vi "P4CMDSub Verify File Status for CheckIn.vi"(6 "operation message":string, 8 "error in (no error)":errorcluster, 10 "files":path[](array[path]), 11 "source control reference in":T1) -> (0 "error out":errorcluster, 2 "files (depot format)":string[](array[string]), 3 "source control reference out":T1, 5 "active changelist":string)   [LabVIEW 2017, in "NI_SCC_P4CMD.lvlib"]
uses:
  <vilib>/SourceControl/Providers/P4CMD/NI_SCC_P4CMD.lvlib
  <vilib>/SourceControl/sccapi/SCCAPI Refnum.ctl
  <vilib>/SourceControl/support/SCCSup Message Strings GLBL.vi
  <vilib>/SourceControl/sccapi/NI_SCC.lvlib
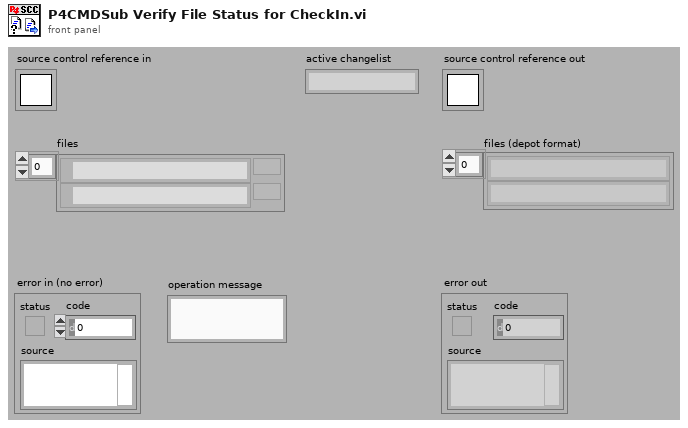
[diagram p1: front panel]
types:
  T1 = typedef "NI_SCC.lvlib/SCCAPI Refnum.ctl" = refnum<k1>
  T2 = typedef "NI_SCC_P4CMD.lvlib/P4CMD SCC File Status.ctl" = cluster{"source controlled":bool, "open by user":bool, "open by other":bool, "out of date":bool, "deleted":bool, "locked by user":bool, "locked by other":bool, "open for add by user":bool, "open for delete by user":bool}
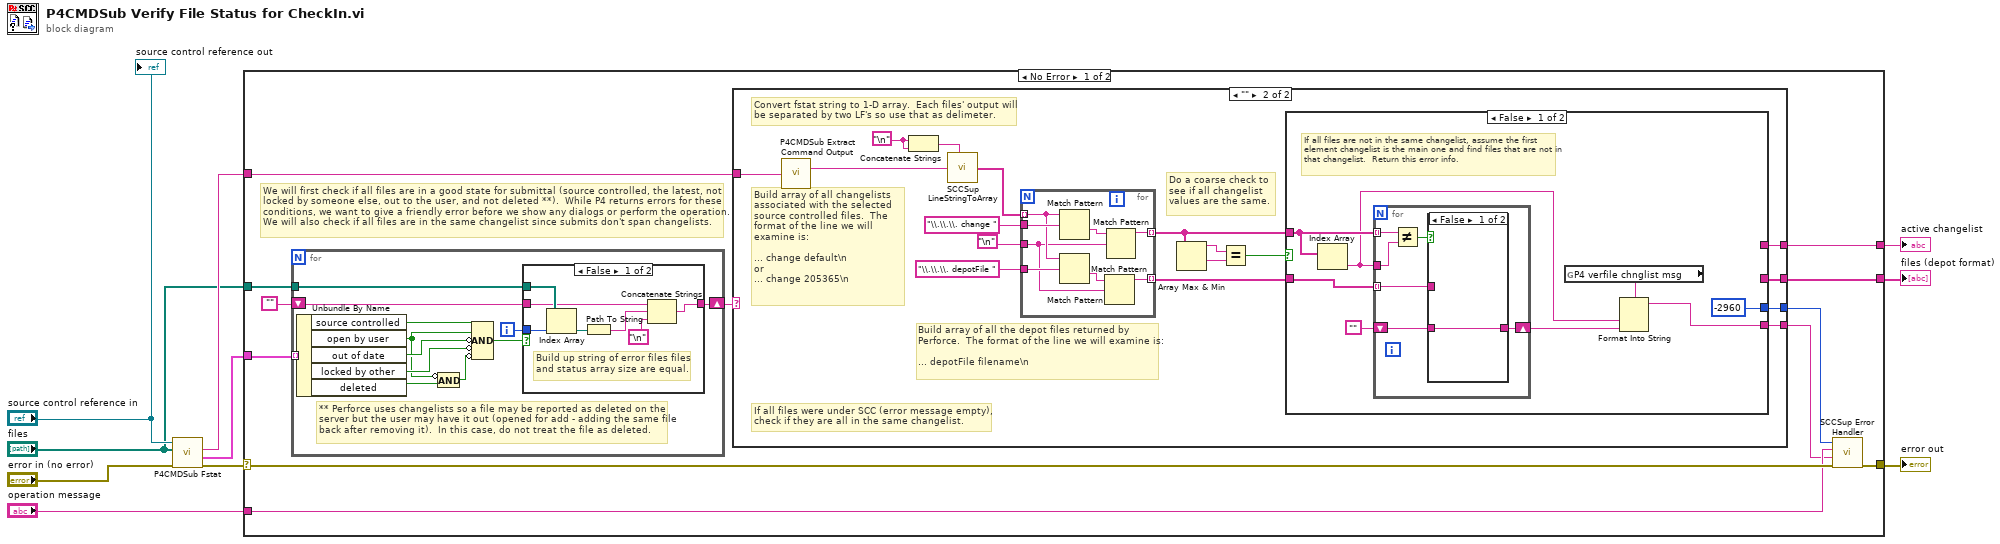
[diagram p0: block diagram]
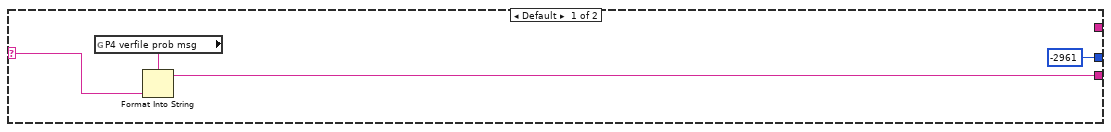
[diagram p2: hidden frame]
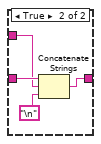
[diagram p3: hidden frame]
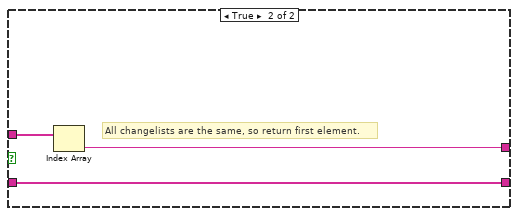
[diagram p4: hidden frame]
diagram:
  n1 = call <vilib>:"P4CMDSub Fstat.vi"("error in (no error)"="error in (no error)", "files"="files", "source control reference in"="source control reference in") -> ("error out"=w8:errorcluster, "files status"=w9:T2[], "fstat output"=w5:string)  [unwired: 5 in, 1 out]
  n2 = case shown="No Error" w8 {
    selector: w8 -> [w21 w94]
    tunnel: w9 -> [w22 _]
    tunnel: [w20 w94] -> w7
    tunnel: w5 -> [w19 _]
    tunnel: [w17 _] -> w4
    tunnel: [w18 _] -> w3
    tunnel: "operation message" -> [w16 _]
    tunnel: "files" -> [w15 _]
    frame No Error {
      # "We will first check if all files are in a good state for submittal (source controlled, the latest, not locked by someone else, out to the user, and not deleted **).  While P4 returns errors for these conditions, we want to give a friendly error before we show any dialogs or perform the operation.  We will also check if all files are in the same changelist since submits don't span changelists."
      n3 = for {
        tunnel: w22 -> [w85] mode=indexing
        tunnel: w15 -> [w84]
        shift-right: [w81] -> w13
        shift-left: "" -> [w82]
        i -> [w83]
        # "** Perforce uses changelists so a file may be reported as deleted on the server but the user may have it out (opened for add - adding the same file back after removing it).  In this case, do not treat the file as deleted."
        n4 = Unbundle By Name(w85) -> ("source controlled"=w80:bool, "open by user"=w76:bool, "out of date"=w79:bool, "locked by other"=w78:bool, "deleted"=w75:bool)
        n5 = Compound Arithmetic op=AND(invert w76, w75) -> (w74:bool)
        n6 = Compound Arithmetic op=AND(w80, w76, invert w79, invert w78, invert w74) -> (w77:bool)
        n7 = case shown="False" w77 {
          tunnel: w84 -> [w92 _]
          tunnel: w83 -> [w91 _]
          tunnel: w82 -> [w90 w93]
          tunnel: [w88 w93] -> w81
          frame False {
            # "Build up string of error files files and status array size are equal."
            n8 = Index Array(array=w92, index=w91) -> (element=w87:path)
            n9 = Path To String(path=w87) -> (string=w86:string)
            n10 = Concatenate Strings(w90, w86, "\n") -> (w88:string)
          }
          frame True {
          }
        }
      }
      n11 = case shown="\"\"" w13 {
        selector: w13 -> [w26 _]
        tunnel: w19 -> [_ w28]
        tunnel: [_ w32] -> w18
        tunnel: [_ w31] -> w17
        tunnel: [w25 w29] -> w11
        tunnel: [-2961 ("error code") w30] -> w12
        frame Default {
          n12 = global read "SCCSup Message Strings GLBL.vi" "P4 verfile prob msg"() -> (w23:string)
          n13 = Format Into String(format string=w23, w26) -> (resulting string=w25:string)  [unwired: 2 in, 1 out]
        }
        frame "" {
          w43 = "\n"
          # "If all files were under SCC (error message empty), check if they are all in the same changelist."
          # "Build array of all the depot files returned by Perforce.  The format of the line we will examine is:\n\n... depotFile filename\\n"
          # "Do a coarse check to see if all changelist values are the same."
          # "Build array of all changelists associated with the selected source controlled files.  The format of the line we will examine is:\n\n... change default\\n\nor\n... change 205365\\n"
          # "Convert fstat string to 1-D array.  Each files' output will be separated by two LF's so use that as delimeter."
          n14 = call <vilib>:"P4CMDSub Extract Command Output.vi"("bundled message"=w28) -> ("command output"=w27:string)  [unwired: 13 in, 1 out]
          n15 = Concatenate Strings(w43, w43) -> (w42:string)
          n16 = call <vilib>:"SCCSup LineStringToArray.vi"("delimiter (Tab)"=w42, "line string"=w27) -> ("line array"=w39:string[])  [unwired: 7 in]
          n17 = for {
            tunnel: "\\.\\.\\. change " ("regular expression") -> [w73]
            tunnel: "\n" -> [w67]
            tunnel: w39 -> [w70] mode=indexing
            tunnel: [w71] -> w33 mode=indexing
            tunnel: "\\.\\.\\. depotFile " ("regular expression") -> [w69]
            tunnel: [w66] -> w34 mode=indexing
            n18 = Match Pattern(string=w70, regular expression=w73) -> (after substring=w72:string)  [unwired: 1 in, 3 out]
            n19 = Match Pattern(string=w70, regular expression=w69) -> (after substring=w68:string)  [unwired: 1 in, 3 out]
            n20 = Match Pattern(string=w68, regular expression=w67) -> (before substring=w66:string)  [unwired: 1 in, 3 out]
            n21 = Match Pattern(string=w72, regular expression=w67) -> (before substring=w71:string)  [unwired: 1 in, 3 out]
          }
          n22 = Array Max & Min(array=w33) -> (max value=w36:string, min value=w38:string)  [unwired: 2 out]
          n23 = Equal?(x=w36, y=w38) -> (x = y?=w35:bool)
          n24 = case shown="False" w35 {
            tunnel: w34 -> [w49 w64]
            tunnel: w33 -> [w50 w65]
            tunnel: [_ w64] -> w32
            tunnel: [_ w63] -> w31
            tunnel: [-2960 ("error code") _] -> w30
            tunnel: [w46 _] -> w29
            frame False {
              # "If all files are not in the same changelist, assume the first element changelist is the main one and find files that are not in that changelist.  Return this error info."
              n25 = Index Array(array=w50) -> (element=w45:string)  [unwired: 1 in]
              n26 = for {
                tunnel: w50 -> [w57] mode=indexing
                tunnel: w49 -> [w53] mode=indexing
                tunnel: w45 -> [w56]
                shift-right: [w52] -> w47
                shift-left: "" -> [w54]
                n27 = Not Equal?(x=w57, y=w56) -> (x != y?=w55:bool)
                n28 = case shown="False" w55 {
                  tunnel: w54 -> [w58 w61]
                  tunnel: w53 -> [_ w60]
                  tunnel: [w58 w59] -> w52
                  frame False {
                  }
                  frame True {
                    n29 = Concatenate Strings(w61, w60, "\n") -> (w59:string)
                  }
                }
              }
              n30 = global read "SCCSup Message Strings GLBL.vi" "P4 verfile chnglist msg"() -> (w44:string)
              n31 = Format Into String(format string=w44, w45, w47) -> (resulting string=w46:string)  [unwired: 2 in, 1 out]
            }
            frame True {
              # "All changelists are the same, so return first element."
              n32 = Index Array(array=w65) -> (element=w63:string)  [unwired: 1 in]
            }
          }
        }
      }
      n33 = call <vilib>:"SCCSup Error Handler.vi"("error in (no error)"=w21, "additional message"=w11, "operation message"=w16, "scc error code"=w12) -> ("error out"=w20:errorcluster)  [unwired: 7 in]
    }
    frame Error {
    }
  }
  "error out" <- w7
  "active changelist" <- w4
  "files (depot format)" <- w3
  "source control reference out" <- "source control reference in"
